vi "Send Response.vi"(8 "error in (no error)":errorcluster, 9 "timeout in ms (0)":i32 format="%d ms", 10 "response":T1, 11 "Plugin Thread in":refnum<class "Plugin Thread.lvclass">) -> (0 "error out":errorcluster, 3 "Plugin Thread out":refnum<class "Plugin Thread.lvclass">)   [LabVIEW 2019, in "DSF Core.lvlib" / "Plugin Thread.lvclass"]
uses:
  Thread/Plugin/Plugin Thread.lvclass
  Interface/Plugin/Response Data.ctl
  Interface/Plugin/Response.ctl
  Interface/Plugin/Response Parameters.ctl
  Thread/Plugin/Plugin Thread.lvclass/Plugin Thread.ctl
  Interface/Interface.lvclass/Interface.ctl
  Interface/Plugin/Send Plugin Response.vi
  Interface/Errors.vi
  Interface/Dispatcher/Response Timeout.vi
  Interface/Plugin/Class Name.vi
  Interface/Write RT FIFO.vi
  Interface/New Interface Error.vi
  <vilib>/NI/Memory Manager/VIs/New Error Cluster.vi
  <vilib>/NI/Memory Manager/VIs/New Error Cluster (512B).vi
  <vilib>/NI/Memory Manager/VIs/Set Error Code.vi
  <vilib>/NI/Memory Manager/VIs/Set Error Status.vi
  <vilib>/NI/Memory Manager/VIs/Set Error Source.vi
  <vilib>/NI/Memory Manager/VIs/Write String to Source.vi
  Interface/Interface Error Info.vi
  VIs/Constants/Constants.vi
  VIs/Constants/Base Error Code.vi
  Interface/Interface Error Offset.vi
  Interface/Plugin/Plugin Interface.lvclass
  C:/Dev/GitHub/niveristand-data-sharing-framework-custom-device/Core/Classes/Interface/Interface.lvclass
  VIs/VI Name.vi
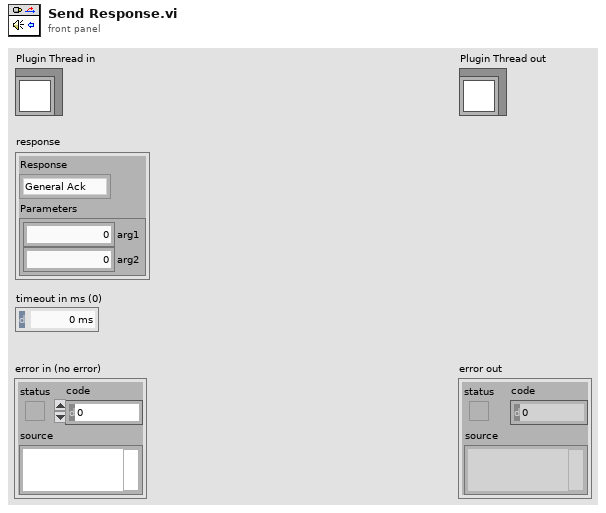
[diagram p1: front panel]
types:
  T1 = typedef "DSF Core.lvlib/Plugin Interface.lvclass/Response Data.ctl" = cluster{"Response":T2, "Parameters":T3}
  T2 = typedef "DSF Core.lvlib/Plugin Interface.lvclass/Response.ctl" = enum8{"General Ack", "Shutting Down"}
  T3 = typedef "DSF Core.lvlib/Plugin Interface.lvclass/Response Parameters.ctl" = cluster{"arg1":u64, "arg2":u64}
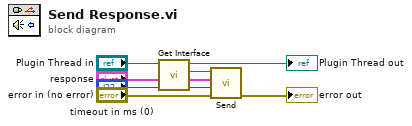
[diagram p0: block diagram]
diagram:
  n1 = call "Get Interface.vi"("Transceiver Thread in"="Plugin Thread in") -> ("Interface"=w6:refnum<class "Plugin Interface.lvclass">, "Transceiver Thread out"=→"Plugin Thread out":refnum<class "Plugin Thread.lvclass">)  [unwired: 9 in]
  n2 = call-poly "Send.vi"("error in (no error)"="error in (no error)", "timeout in ms (0)"="timeout in ms (0)", "response"="response", "Plugin Interface in"=w6) -> ("error out"=→"error out":errorcluster)  [unwired: 6 in, 1 out]
